vi "Obtain Default Broadcast Events.vi"(8 "error in (no error)":errorcluster) -> (0 "error out":errorcluster, 1 "Update Module Execution Status":refnum<user-event>, 2 "Error Reported":refnum<user-event>, 3 "Status Updated":refnum<user-event>, 4 "System Message":refnum<user-event>, 5 "Module Did Stop":refnum<user-event>)   [LabVIEW 2020, in "ActorModule.lvlib"]
doc: "This a wrapper VI for the Obtain Broadcast Events for Registration.vi. By stripping the module-specific controls from its terminals and facilitating a default connector pane, it enables the startup.vi to register for the common events (Status, Error, Stop, Execution Status) dynamically (without static linking).\n\n____\nHAMPEL SOFTWARE ENGINEERING v2.6.0 (2023-12-19 10:54)"
uses:
  ActorModule.lvlib
  Status Updated Argument--cluster.ctl
  Error Reported Argument--cluster.ctl
  Stop Argument--cluster.ctl
  Get Module Execution Status Argument--cluster.ctl
  System Message Argument--cluster.ctl
  Libraries/hse-libraries/Source/hse-dqmh/Controls/System Message Source.ctl
  Libraries/hse-libraries/Source/hse-dqmh/hse-dqmh.lvlib
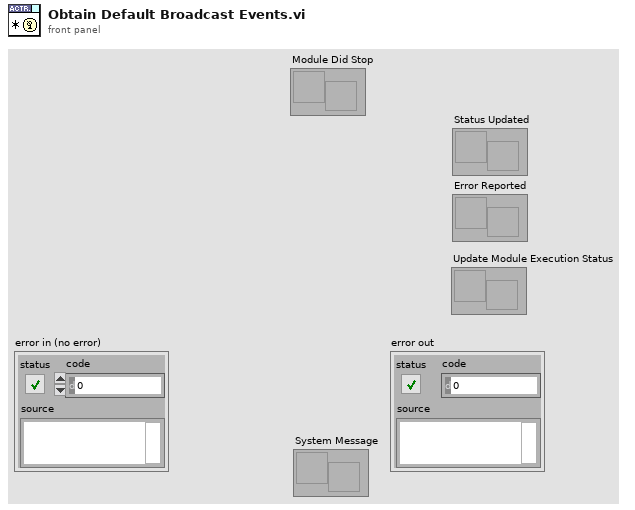
[diagram p1: front panel]
types:
  T1 = typedef "ActorModule.lvlib/Broadcast Events--cluster.ctl" = cluster{"Module Did Init":refnum<user-event>, "Status Updated":refnum<user-event>, "Error Reported":refnum<user-event>, "Module Did Stop":refnum<user-event>, "Update Module Execution Status":refnum<user-event>, "System Message":refnum<user-event>}
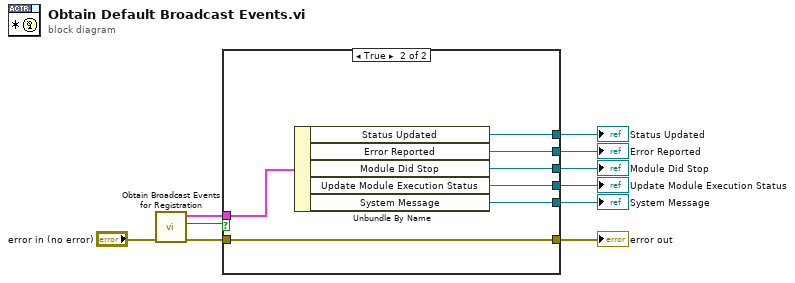
[diagram p0: block diagram]
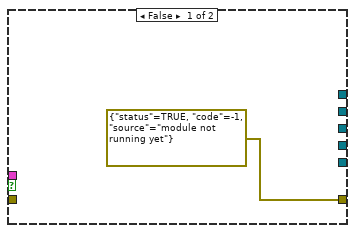
[diagram p2: hidden frame]
diagram:
  n1 = call "Obtain Broadcast Events for Registration.vi"("error in (no error)"="error in (no error)") -> ("error out"=w9:errorcluster, "Already running?"=w6:bool, "ActorModule Broadcast Events"=w7:T1)  [unwired: 8 in]
  n2 = case shown="True" w6 {
    tunnel: w7 -> [_ w18]
    tunnel: [errorcluster {"status"=TRUE, "code"=-1, "source"="module not running yet"} ("error out") w17] -> w10
    tunnel: w9 -> [_ w17]
    tunnel: [_ w16] -> w5
    tunnel: [_ w15] -> w4
    tunnel: [_ w14] -> w3
    tunnel: [_ w13] -> w2
    tunnel: [_ w12] -> w1
    frame False {
    }
    frame True {
      n3 = Unbundle By Name(w18) -> ("Status Updated"=w16:refnum<user-event>, "Error Reported"=w15:refnum<user-event>, "Module Did Stop"=w14:refnum<user-event>, "Update Module Execution Status"=w13:refnum<user-event>, "System Message"=w12:refnum<user-event>)
    }
  }
  "error out" <- w10
  "Status Updated" <- w5
  "Error Reported" <- w4
  "Module Did Stop" <- w3
  "Update Module Execution Status" <- w2
  "System Message" <- w1
